vi "UDPrecieverMin.vi"() -> ()   [LabVIEW 2012]
panel:
  out "Raw Data Out":string
  out "error post-check":errorcluster
  out "End Reciever Error":errorcluster
  in  "stop reciever":bool
  out "port":u16
  out "error out post-read":errorcluster
  out "error out pre-read":errorcluster
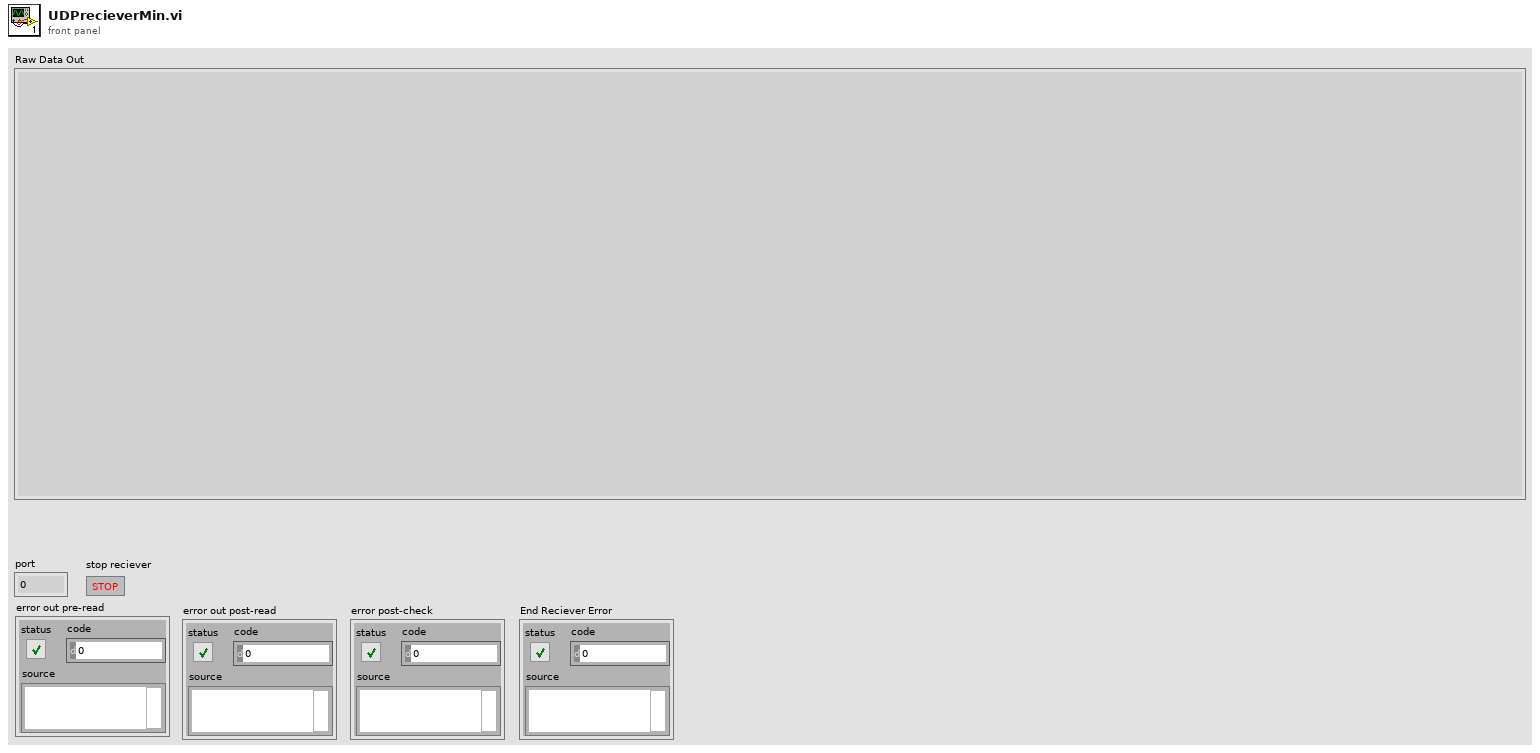
[diagram p1: front panel]
types:
  T1 = enum16{"open", "replace", "create", "open or create", "replace or create", "replace or create with confirmation"}
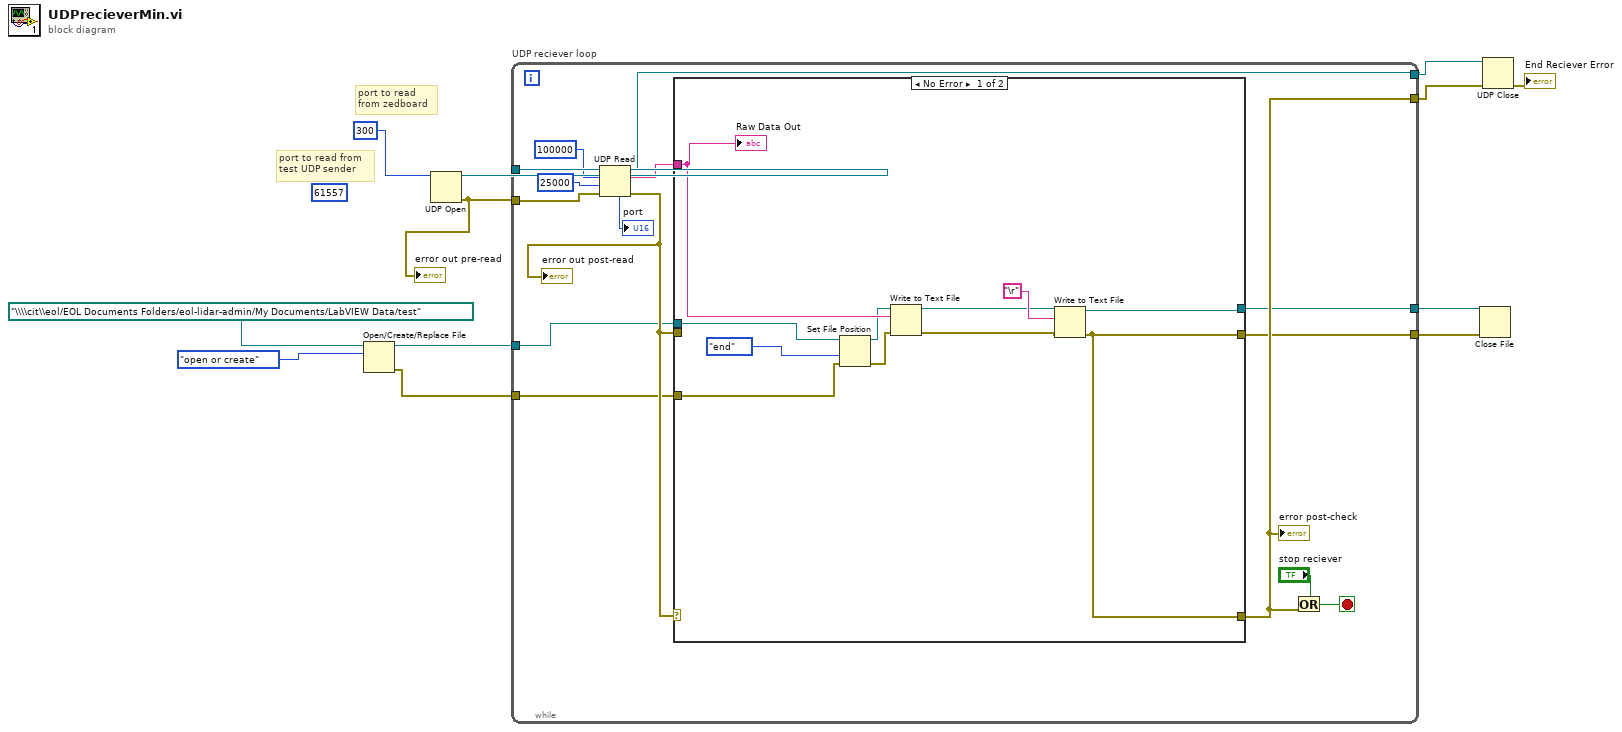
[diagram p0: block diagram]
diagram:
  (unwired) u16 61557 ("port")
  # "port to read \nfrom zedboard"
  # "port to read from \ntest UDP sender"
  n1 = Open/Create/Replace File(file path (use dialog)=path "\\\\cit\\eol/EOL Documents Folders/eol-lidar-admin/My Documents/LabVIEW Data/test" ("file (use dialog)"), operation (0:open)=T1."open or create") -> (refnum out=w5:refnum<file>, error out=w3:errorcluster)  [unwired: 4 in, 1 out]
  n2 = UDP Open(11:u16 300 ("port")) -> (port=w11:refnum<k16>, 0:w8:errorcluster)  [unwired: 4 in, 1 out]
  "error out pre-read" <- w8
  n3 = while "UDP reciever loop" {
    tunnel: [w27] -> w12
    tunnel: w11 -> [w26]
    tunnel: [w19] -> w10
    tunnel: w8 -> [w23]
    tunnel: w5 -> [w16]
    tunnel: w3 -> [w15]
    tunnel: [w14] -> w2
    tunnel: [w13] -> w1
    stop <- w25 stop-if-true
    n4 = UDP Read(connection ID=w26, max size (548)=100000, timeout ms (25000)=25000, 8:w23) -> (data out=w21:string, error out=w17:errorcluster, 3:w27:refnum<k16>, 4:→"port":u16)  [unwired: 1 out]
    "error out post-read" <- w17
    n5 = case shown="No Error" w17 {
      selector: w17 -> [_ w41]
      tunnel: w21 -> [w38 _]
      tunnel: [w29 w41] -> w19
      tunnel: w17 -> [_ _]
      tunnel: w16 -> [w34 w40]
      tunnel: w15 -> [w33 w39]
      tunnel: [w29 w39] -> w14
      tunnel: [w28 w40] -> w13
      frame No Error {
        n6 = Set File Position(refnum=w34, from (0:start)=enum16{"start", "end", "current"}."end", error in=w33) -> (refnum out=w35:refnum<file>, error out=w36:errorcluster)  [unwired: 1 in]
        n7 = Write to Text File(file (use dialog)=w35, text=w38, error in=w36) -> (refnum out=w31:refnum<file>, error out=w30:errorcluster)  [unwired: 1 in, 1 out]
        n8 = Write to Text File(file (use dialog)=w31, text="\r", error in=w30) -> (refnum out=w28:refnum<file>, error out=w29:errorcluster)  [unwired: 1 in, 1 out]
        "Raw Data Out" <- w38
      }
      frame Error {
      }
    }
    "error post-check" <- w19
    n9 = Or(x="stop reciever", y=w19) -> (x .or. y?=w25:bool)
  }
  n10 = Close File(refnum=w1, error in=w2) -> ()  [unwired: 2 out]
  n11 = UDP Close(connection ID=w12, 8:w10) -> (error out=→"End Reciever Error":errorcluster)  [unwired: 1 out]
